vi "test_maxSearch.vi"() -> ()   [LabVIEW 2016]
uses:
  <vilib>/rvi/DesktopExecutionNode/Execution/niFpgaDEN_Execute.vi
  <vilib>/rvi/DesktopExecutionNode/DesktopExecutionNode.xnode
panel:
  out "validPoints":cluster{"index":u16, "data":i16, i32}[](array[cluster])
  out "Array 2":bool[](array[boolean])
  out "Array":T1(array[cluster])
  out "dataIn":dbl[](graph)
  in  "numTicks":i32
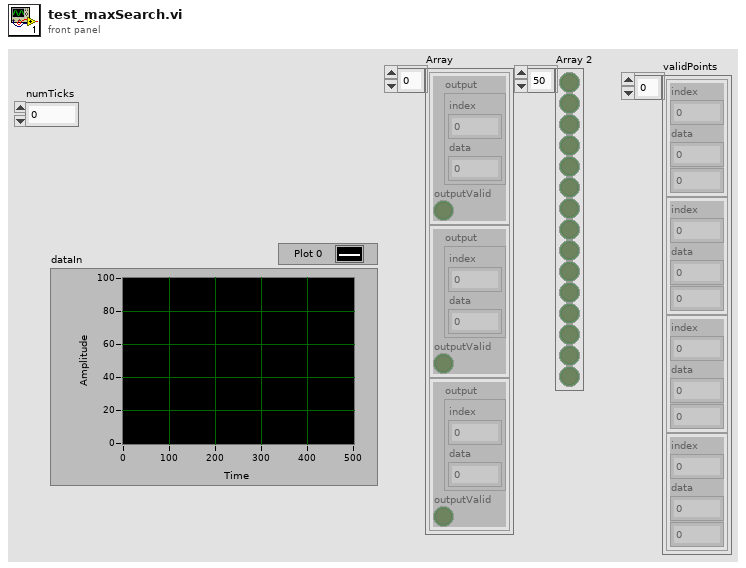
[diagram p1: front panel]
types:
  T1 = cluster{"output":cluster{"index":u16, "data":i16}, "outputValid":bool}[]
  T2 = cluster{"maxSearchUpper":u16, "maxSearchLower":u16}
  T3 = cluster{"output":cluster{"index":u16, "data":i16}, "outputValid":bool}
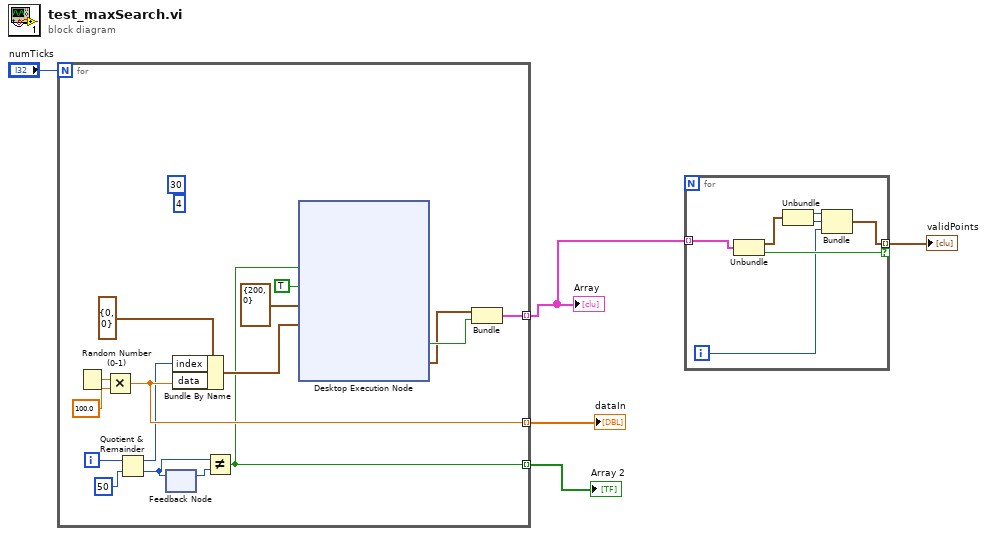
[diagram p0: block diagram]
diagram:
  n1 = for {
    N: "numTicks" -> [_]
    tunnel: [w16] -> w2 mode=indexing
    tunnel: [w15] -> w4 mode=indexing
    tunnel: [w7] -> w3 mode=indexing
    i -> [w18]
    (unwired) u16 30 ("syncPoint")
    (unwired) u16 4 ("syncAverageBand")
    n2 = Random Number (0-1)() -> (number: 0 to 1=w20:dbl)
    n3 = Multiply(x=w20, y=100.0) -> (x*y=w15:dbl)
    n4 = Quotient & Remainder(x=w18, y=50) -> (x-y*floor(x/y)=w8:i32, floor(x/y)=w6:i32)
    n5 = feedback-in #1(w6) -> ()
    n6 = feedback #1() -> (w9:i32)  [unwired: 1 in]
    n7 = Bundle By Name(cluster=cluster{"index":u16, "data":i16} {"index"=0, "data"=0} ("input"), "index"=w8, "data"=w15) -> (w14:cluster{"index":u16, "data":i16})
    n8 = Not Equal?(x=w6, y=w9) -> (x != y?=w7:bool)
    n9 = xnode "Desktop Execution Node"("reset"=w7, "enable"=TRUE, "maxSearchBounds"=T2 {"maxSearchUpper"=200, "maxSearchLower"=0}, "inputPair"=w14) -> ("outputValid"=w11:bool, "output"=w10:cluster{"index":u16, "data":i16})  [unwired: 1 in, 1 out]
    n10 = Bundle("output"=w10, "outputValid"=w11) -> (w16:T3)  [unwired: 1 in]
  }
  "dataIn" <- w4
  "Array" <- w2
  "Array 2" <- w3
  n11 = for {
    tunnel: w2 -> [w28] mode=indexing
    tunnel: [w22] -> w1 mode=indexing if=w27
    i -> [w23]
    n12 = Unbundle(w28) -> ("output"=w26:cluster{"index":u16, "data":i16}, "outputValid"=w27:bool)
    n13 = Unbundle(w26) -> ("index"=w25:u16, "data"=w24:i16)
    n14 = Bundle("index"=w25, "data"=w24, w23) -> (w22:cluster{"index":u16, "data":i16, i32})  [unwired: 1 in]
  }
  "validPoints" <- w1
